vi "SetOptionTest.vi"() -> ()   [LabVIEW 2025]
uses:
  common/ClientNetworkInterfaceGlobalVariables.vi
panel:
  out "Sent Message":string
  in  "Option":string
  out "Return Message":string
  in  "Value":dbl=1.0 min=0.0 max=1.0 step=0.1
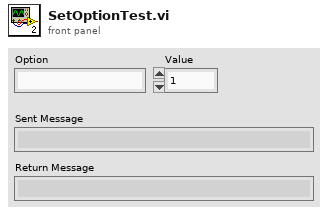
[diagram p1: front panel]
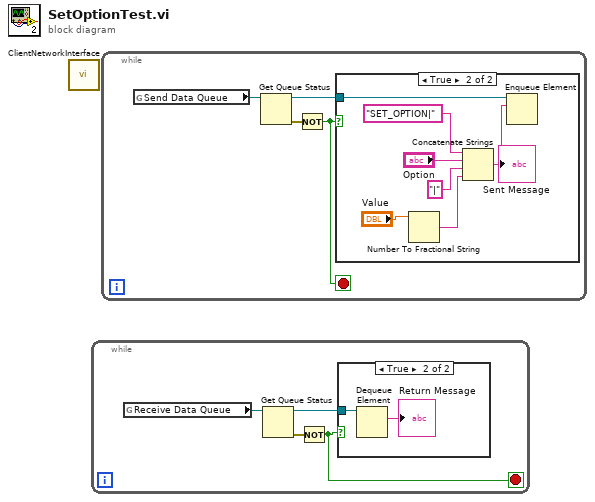
[diagram p0: block diagram]
diagram:
  n1 = call "ClientNetworkInterface.vi"() -> ()  [unwired: 1 in]
  n2 = while {
    stop <- w1 stop-if-true
    n3 = global read "ClientNetworkInterfaceGlobalVariables.vi" "Receive Data Queue"() -> (w4:refnum<queue>)
    n4 = Get Queue Status(queue=w4) -> (queue out=w3:refnum<queue>, error out=w2:errorcluster)  [unwired: 2 in, 6 out]
    n5 = Not(x=w2) -> (.not. x?=w1:bool)
    n6 = case shown="True" w1 {
      tunnel: w3 -> [_ w5]
      frame False {
      }
      frame True {
        n7 = Dequeue Element(queue=w5) -> (element=→"Return Message":string)  [unwired: 2 in, 3 out]
      }
    }
  }
  n8 = while {
    stop <- w7 stop-if-true
    n9 = global read "ClientNetworkInterfaceGlobalVariables.vi" "Send Data Queue"() -> (w10:refnum<queue>)
    n10 = Get Queue Status(queue=w10) -> (queue out=w9:refnum<queue>, error out=w8:errorcluster)  [unwired: 2 in, 6 out]
    n11 = Not(x=w8) -> (.not. x?=w7:bool)
    n12 = case shown="True" w7 {
      tunnel: w9 -> [_ w16]
      frame False {
      }
      frame True {
        n13 = Number To Fractional String(number="Value") -> (F-format string=w12:string)  [unwired: 3 in]
        n14 = Concatenate Strings("SET_OPTION|" ("string"), "Option", "|" ("string"), w12) -> (w11:string)
        "Sent Message" <- w11
        n15 = Enqueue Element(queue=w16, element=w11) -> ()  [unwired: 2 in, 3 out]
      }
    }
  }
